vi "flight_time_05_12_v3.vi"() -> ()   [LabVIEW 2013]
uses:
  <vilib>/Instr/_visa.llb/VISA Configure Serial Port (Instr).vi
  <vilib>/Analysis/NI_AALBase.lvlib
panel:
  in  "flight_h_store":u32[](array[numeric])
  in  "flight_time_store":u32[](array[numeric])
  in  "lock":u8=3
  out "avg_cell4":dbl
  out "avg_cell3":dbl
  out "avg_cell2":dbl
  out "avg_cell1":dbl
  in  "stop":bool
  in  "Pcell1":u32[](array[numeric])
  in  "Pcell2":u32[](array[numeric])
  in  "Pcell3":u32[](array[numeric])
  in  "Pcell4":u32[](array[numeric])
  in  "Tab Control":enum32{"Calibração", "filter"}(tab)
  out "raw_cell1":dbl(graph) caption="Celula 1"
  out "raw_cell2":dbl(graph) caption="Celula 2"
  out "raw_cell3":dbl(graph) caption="Celula 3"
  out "raw_cell4":dbl(graph) caption="Celula 4"
  out "flight_h_graph":u32[](graph) caption="flight_time_graph"
  out "state":bool
  out "calibrado1":dbl(graph) caption="Celula 1"
  out "calibrado3":dbl(graph) caption="Celula 3"
  out "calibrado2":dbl(graph) caption="Celula 2"
  out "calibrado4":dbl(graph) caption="Celula 4"
  in  "?":bool
  out "tempo de voo ultimo pulo (ms)":dbl
  in  "?":bool
  out "h":dbl caption="Altura ultimo pulo (cm)"
  out "fEq":dbl(graph)
  out "flight_time_graph":u32[](graph)
  out "cell":u8[](array[numeric])
  out "output_int16":i32[](array[numeric])
  out "data":u8[](array[numeric])
  in  "serial_port":refnum<visa-resource-name>="COM7" caption="Porta Serial"
  # "Aguarde 10 segundos para a calibração do sistema"
  # "Sistema calibrado e pronto para operação"
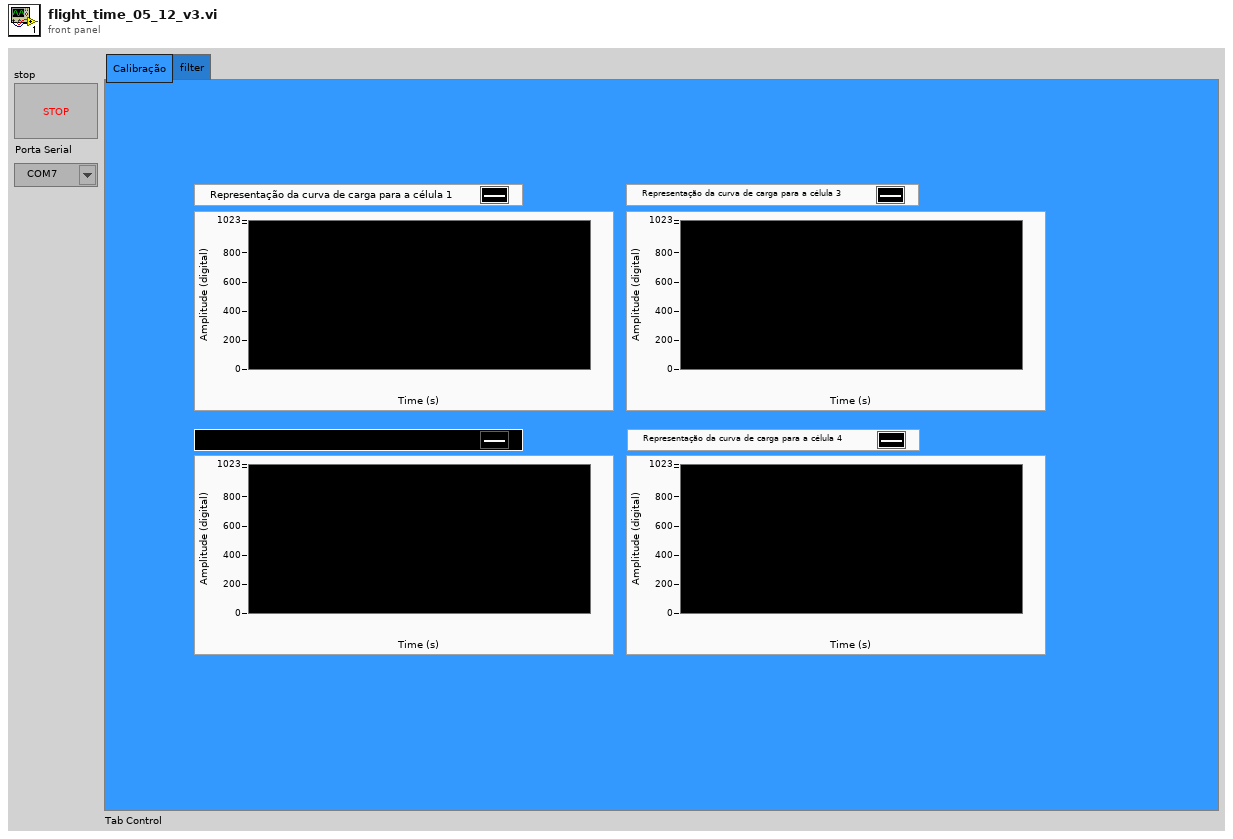
[diagram p1: front panel]
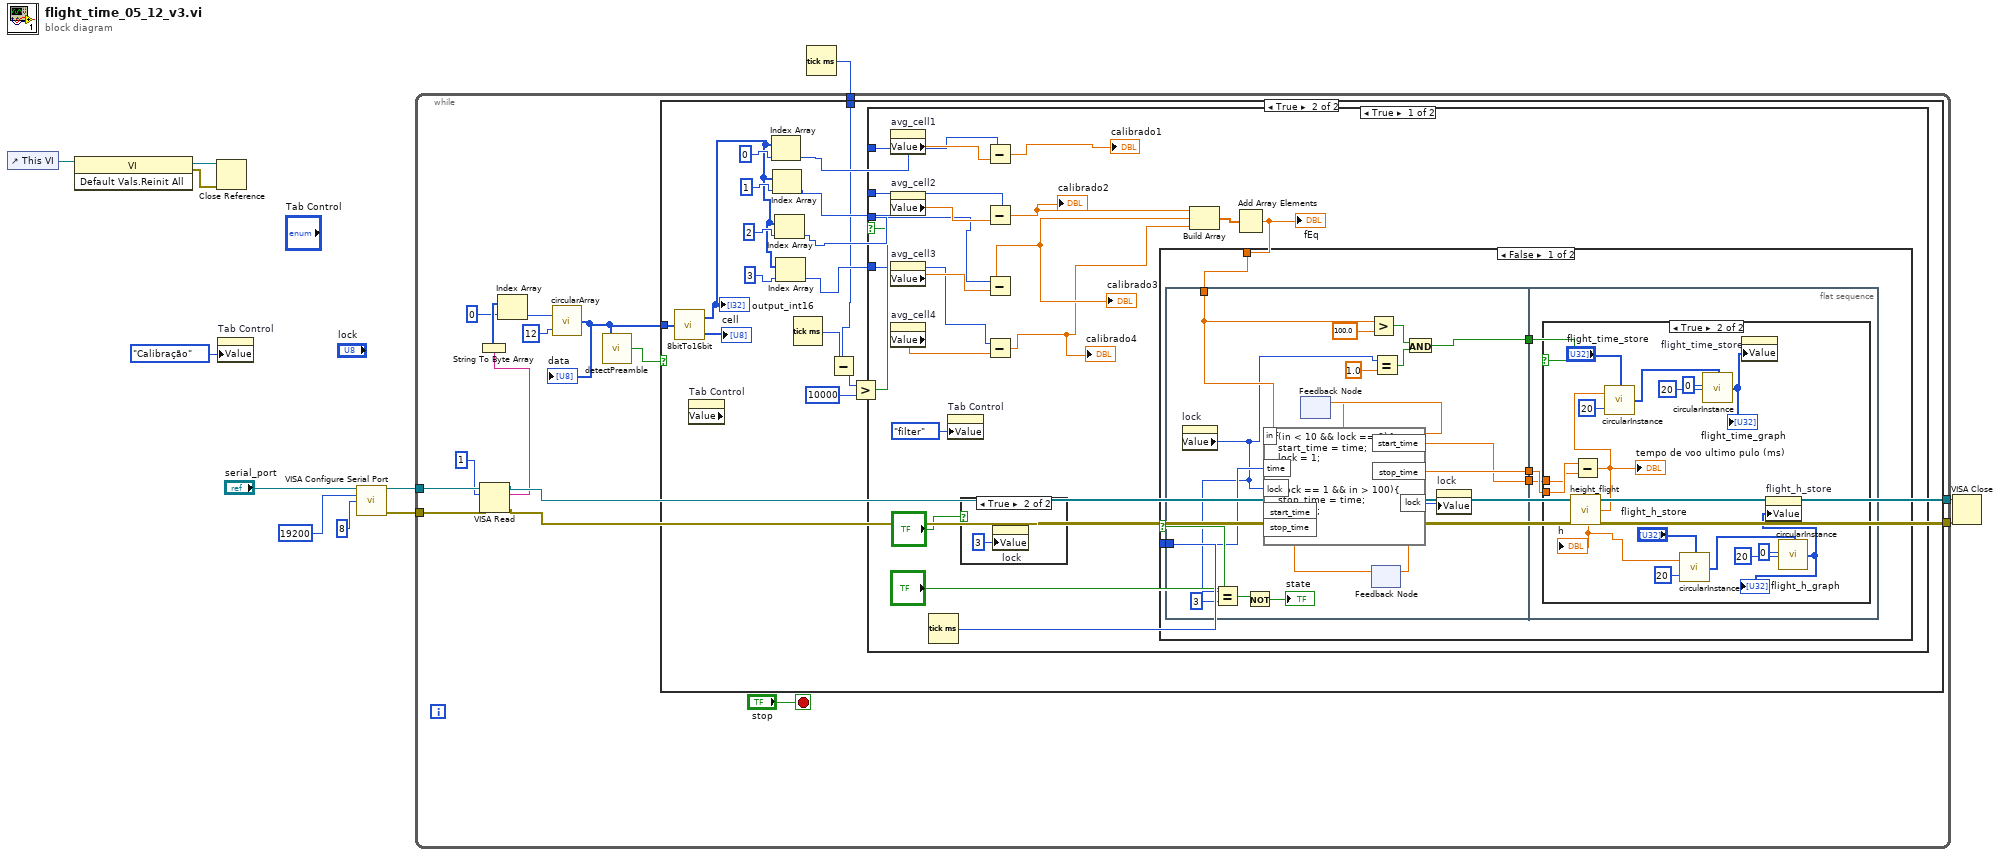
[diagram p0: block diagram]
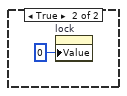
[diagram p5: hidden frame]
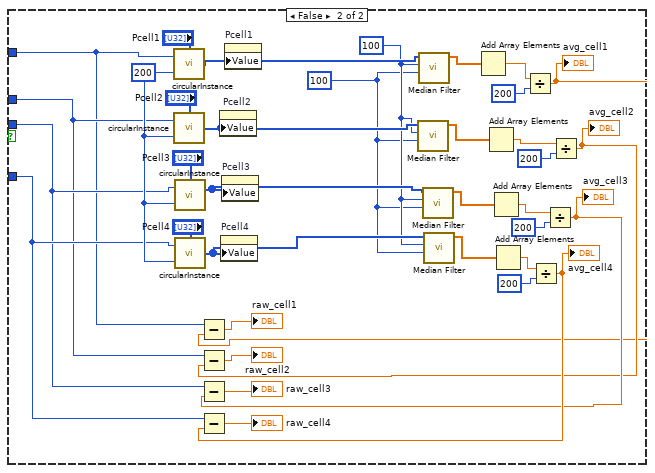
[diagram p6: hidden frame]
diagram:
  n1 = control-ref of="This VI"() -> (w3:refnum<vi>)
  n2 = invoke class="VI" method="Default Vals.Reinit All"(reference=w3) -> (reference out=w2:refnum<vi>, error out=w1:errorcluster)  [unwired: 2 in, 1 out]
  n3 = Close Reference(reference=w2, error in (no error)=w1) -> ()  [unwired: 1 out]
  n4 = property on="Tab Control" class="TabCtl (strict)"("Value"=enum32{"Calibração", "filter"}."Calibração" ("Tab Control")) -> ()  [unwired: 2 in, 2 out]
  n5 = call-poly "VISA Configure Serial Port"("VISA resource name"="serial_port", "baud rate (9600)"=u32 19200, "data bits (8)"=u16 8) -> ("VISA resource name out"=w9:refnum<visa-resource-name>, "error out"=w8:errorcluster)  [unwired: 11 in]
  n6 = Tick Count (ms)() -> (millisecond timer value=w5:u32)
  n7 = while {
    tunnel: w9 -> [w26]
    tunnel: w8 -> [w25]
    tunnel: [w23] -> w6
    tunnel: [w24] -> w7
    tunnel: w5 -> [w13]
    stop <- "stop" stop-if-true
    n8 = VISA Read(VISA resource name=w26, byte count=1, error in (no error)=w25) -> (VISA resource name out=w24:refnum<visa-resource-name>, read buffer=w18:string, error out=w23:errorcluster)  [unwired: 1 out]
    n9 = String To Byte Array(string=w18) -> (unsigned byte array=w21:u8[])
    n10 = Index Array(array=w21, index=0) -> (element=w15:u8)
    n11 = call "circularArray.vi"("max-size"=u8 12, "element"=w15) -> ("dataout"=w16:u8[])
    "data" <- w16
    n12 = call "detectPreamble.vi"("data-in"=w16) -> ("detected"=w14:bool)
    n13 = case shown="True" w14 {
      tunnel: w16 -> [_ w41]
      tunnel: w13 -> [_ w30]
      frame False {
      }
      frame True {
        n14 = call "8bitTo16bit.vi"("input_byte"=w41) -> ("output_int16"=w36:i32[], "cell"=→"cell":u8[])
        "output_int16" <- w36
        n15 = property on="Tab Control" class="TabCtl (strict)" props=["Value"]() -> ()  [unwired: 2 in, 3 out]
        n16 = Index Array(array=w36, index=0) -> (element=w32:i32)
        n17 = Index Array(array=w36, index=1) -> (element=w33:i32)
        n18 = Index Array(array=w36, index=2) -> (element=w34:i32)
        n19 = Index Array(array=w36, index=3) -> (element=w35:i32)
        n20 = Tick Count (ms)() -> (millisecond timer value=w31:u32)
        n21 = Subtract(x=w31, y=w30) -> (x-y=w29:u32)
        n22 = Greater?(x=w29, y=u32 10000) -> (0:w27:bool)
        n23 = case shown="True" w27 {
          tunnel: w32 -> [w53 w106]
          tunnel: w33 -> [w50 w107]
          tunnel: w34 -> [w51 w108]
          tunnel: w35 -> [w52 w114]
          frame True {
            n24 = property on="avg_cell1" class="DigNum (strict)"() -> ("Value"=w58:dbl)  [unwired: 2 in, 2 out]
            n25 = property on="avg_cell2" class="DigNum (strict)"() -> ("Value"=w57:dbl)  [unwired: 2 in, 2 out]
            n26 = property on="avg_cell3" class="DigNum (strict)"() -> ("Value"=w56:dbl)  [unwired: 2 in, 2 out]
            n27 = property on="avg_cell4" class="DigNum (strict)"() -> ("Value"=w55:dbl)  [unwired: 2 in, 2 out]
            n28 = Tick Count (ms)() -> (millisecond timer value=w60:u32)
            n29 = property on="Tab Control" class="TabCtl (strict)"("Value"=enum32{"Calibração", "filter"}."filter" ("Tab Control")) -> ()  [unwired: 2 in, 2 out]
            n30 = case shown="True" "?" {
              frame False {
              }
              frame True {
                n31 = property on="lock" class="DigNum (strict)"("Value"=u8 3 ("lock")) -> ()  [unwired: 2 in, 2 out]
              }
            }
            n32 = Subtract(x=w53, y=w58) -> (x-y=→"calibrado1":dbl)
            n33 = Subtract(x=w50, y=w57) -> (x-y=w48:dbl)
            "calibrado2" <- w48
            n34 = Subtract(x=w51, y=w56) -> (x-y=w47:dbl)
            "calibrado3" <- w47
            n35 = Subtract(x=w52, y=w55) -> (x-y=w46:dbl)
            "calibrado4" <- w46
            n36 = Build Array(w48, w47, w46) -> (w54:dbl[])
            n37 = Add Array Elements(numeric array=w54) -> (sum=w43:dbl)
            "fEq" <- w43
            n38 = case shown="False" "?" {
              tunnel: w60 -> [w66 _]
              tunnel: w43 -> [w65 _]
              frame False {
                n39 = flat-sequence {
                  tunnel: w66 -> [w82]
                  tunnel: w65 -> [w75]
                  tunnel: [w69] -> w64
                  tunnel: [w68] -> w63
                  tunnel: [w67] -> w62
                  tunnel: w64 -> [w83]
                  tunnel: w63 -> [w85]
                  tunnel: w62 -> [w84]
                  frame #0 {
                    n40 = property on="lock" class="DigNum (strict)"() -> ("Value"=w72:u8)  [unwired: 2 in, 2 out]
                    n41 = Equal?(x=w72, y=u8 3) -> (x = y?=w77:bool)
                    n42 = Not(x=w77) -> (.not. x?=→"state":bool)
                    n43 = feedback #1() -> (w79:dbl)  [unwired: 1 in]
                    n44 = Greater?(x=w75, y=100.0) -> (0:w70:bool)
                    n45 = feedback #2() -> (w80:dbl)  [unwired: 1 in]
                    n46 = formula code="if(in < 10 && lock == 0){\n  start_time = time;\n  lock = 1;\n}\n\nif(lock == 1 && in > 100){\n  stop_time = time;\n  lock = 0;\n}"("in"=w75, "time"=w82, "lock"=w72, "start_time"=w79, "stop_time"=w80) -> ("start_time"=w67:dbl, "stop_time"=w68:dbl, "lock"=w81:u8)
                    n47 = feedback-in #1(w67) -> ()
                    n48 = feedback-in #2(w68) -> ()
                    n49 = Equal?(x=w72, y=1.0) -> (x = y?=w71:bool)
                    n50 = And(x=w70, y=w71) -> (x .and. y?=w69:bool)
                    n51 = property on="lock" class="DigNum (strict)"("Value"=w81) -> ()  [unwired: 2 in, 2 out]
                  }
                  frame #1 {
                    n52 = case shown="True" w83 {
                      tunnel: w85 -> [_ w99]
                      tunnel: w84 -> [_ w98]
                      frame False {
                      }
                      frame True {
                        n53 = Subtract(x=w99, y=w98) -> (x-y=w89:dbl)
                        "tempo de voo ultimo pulo (ms)" <- w89
                        n54 = call "height_flight.vi"("t"=w89) -> ("h"=w86:dbl)
                        "h" <- w86
                        n55 = call "circularInstance.vi"("data"="flight_time_store", "max-size"=i16 20, "element"=w89) -> ("dataout"=w95:u32[])
                        n56 = call "circularInstance.vi"("data"="flight_h_store", "max-size"=i16 20, "element"=w86) -> ("dataout"=w90:u32[])
                        n57 = call "circularInstance.vi"("data"=w95, "max-size"=i16 20, "element"=u32 0) -> ("dataout"=w94:u32[])
                        "flight_time_graph" <- w94
                        n58 = property on="flight_time_store" class="Arr (strict)"("Value"=w94) -> ()  [unwired: 2 in, 2 out]
                        n59 = call "circularInstance.vi"("data"=w90, "max-size"=i16 20, "element"=u32 0) -> ("dataout"=w87:u32[])
                        "flight_h_graph" <- w87
                        n60 = property on="flight_h_store" class="Arr (strict)"("Value"=w87) -> ()  [unwired: 2 in, 2 out]
                      }
                    }
                  }
                }
              }
              frame True {
                n61 = property on="lock" class="DigNum (strict)"("Value"=u8 0 ("input variable")) -> ()  [unwired: 2 in, 2 out]
              }
            }
          }
          frame False {
            w127 = 100 ("left rank")
            w128 = 100 ("left rank")
            w135 = i16 200 ("max-size")
            n62 = call "circularInstance.vi"("data"="Pcell1", "max-size"=w135, "element"=w106) -> ("dataout"=w132:u32[])
            n63 = call "circularInstance.vi"("data"="Pcell2", "max-size"=w135, "element"=w107) -> ("dataout"=w131:u32[])
            n64 = call "circularInstance.vi"("data"="Pcell3", "max-size"=w135, "element"=w108) -> ("dataout"=w130:u32[])
            n65 = call "circularInstance.vi"("data"="Pcell4", "max-size"=w135, "element"=w114) -> ("dataout"=w129:u32[])
            n66 = property on="Pcell2" class="Arr (strict)"("Value"=w131) -> ()  [unwired: 2 in, 2 out]
            n67 = property on="Pcell4" class="Arr (strict)"("Value"=w129) -> ()  [unwired: 2 in, 2 out]
            n68 = property on="Pcell3" class="Arr (strict)"("Value"=w130) -> ()  [unwired: 2 in, 2 out]
            n69 = property on="Pcell1" class="Arr (strict)"("Value"=w132) -> ()  [unwired: 2 in, 2 out]
            n70 = call <vilib>:"Median Filter.vi"("right rank"=w127, "left rank"=w128, "X"=w131) -> ("Filtered X"=w126:dbl[])  [unwired: 7 in, 1 out]
            n71 = call <vilib>:"Median Filter.vi"("right rank"=w127, "left rank"=w128, "X"=w132) -> ("Filtered X"=w116:dbl[])  [unwired: 7 in, 1 out]
            n72 = call <vilib>:"Median Filter.vi"("right rank"=w127, "left rank"=w128, "X"=w130) -> ("Filtered X"=w125:dbl[])  [unwired: 7 in, 1 out]
            n73 = call <vilib>:"Median Filter.vi"("right rank"=w127, "left rank"=w128, "X"=w129) -> ("Filtered X"=w115:dbl[])  [unwired: 7 in, 1 out]
            n74 = Add Array Elements(numeric array=w116) -> (sum=w123:dbl)
            n75 = Add Array Elements(numeric array=w126) -> (sum=w117:dbl)
            n76 = Add Array Elements(numeric array=w125) -> (sum=w118:dbl)
            n77 = Add Array Elements(numeric array=w115) -> (sum=w119:dbl)
            n78 = Divide(x=w123, y=i16 200 ("max-size")) -> (x/y=w109:dbl)
            "avg_cell1" <- w109
            n79 = Subtract(x=w106, y=w109) -> (x-y=→"raw_cell1":dbl)
            n80 = Divide(x=w119, y=i16 200 ("max-size")) -> (x/y=w113:dbl)
            "avg_cell4" <- w113
            n81 = Subtract(x=w114, y=w113) -> (x-y=→"raw_cell4":dbl)
            n82 = Divide(x=w118, y=i16 200 ("max-size")) -> (x/y=w111:dbl)
            "avg_cell3" <- w111
            n83 = Subtract(x=w108, y=w111) -> (x-y=→"raw_cell3":dbl)
            n84 = Divide(x=w117, y=i16 200 ("max-size")) -> (x/y=w110:dbl)
            "avg_cell2" <- w110
            n85 = Subtract(x=w107, y=w110) -> (x-y=→"raw_cell2":dbl)
          }
        }
      }
    }
  }
  n86 = VISA Close(VISA resource name=w7, error in (no error)=w6) -> ()  [unwired: 1 out]
